vi "Execute.vi"(8 "error in (no error)":errorcluster, 10 "Abstract Consumer in":refnum<class "Abstract Consumer.lvclass">, 11 "Log Close Message in":refnum<class "Log Close Message.lvclass">) -> (0 "error out":errorcluster, 1 "Abstract Response out":refnum<class "Abstract Response Message.lvclass">, 2 "Abstract Consumer out":refnum<class "Abstract Consumer.lvclass">, 3 "Log Close Message out":refnum<class "Log Close Message.lvclass">, 4 "Stop?":bool)   [LabVIEW 2020, in "Log Close Message.lvclass"]
uses:
  Log Close Message.lvclass
  Abstract Log Consumer/Abstract Log Consumer.lvclass
  Consumer/Abstract Consumer/Abstract Consumer.lvclass
  Message/Abstract Response Message/Abstract Response Message.lvclass
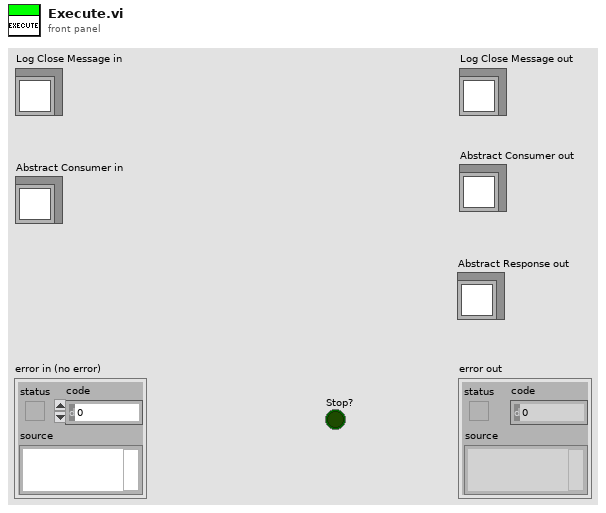
[diagram p1: front panel]
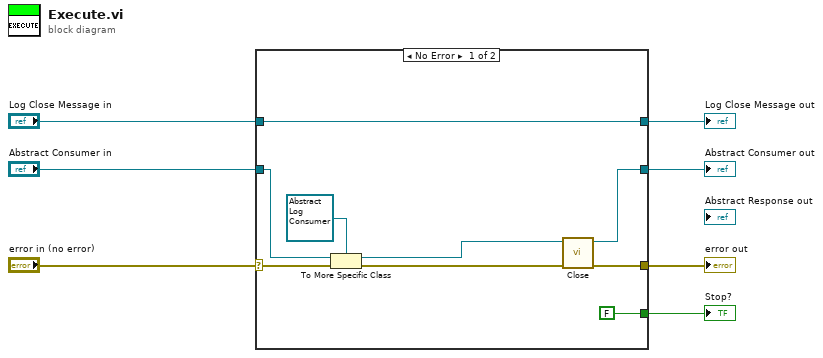
[diagram p0: block diagram]
diagram:
  n1 = case shown="No Error" "error in (no error)" {
    selector: "error in (no error)" -> [w15 w17]
    tunnel: "Abstract Consumer in" -> [w16 w18]
    tunnel: "Log Close Message in" -> [w9 w19]
    tunnel: [w11 w17] -> w4
    tunnel: [w9 w19] -> w2
    tunnel: [w10 w18] -> w1
    tunnel: [FALSE _] -> w3
    frame No Error {
      n2 = To More Specific Class(target class=refnum<class "Abstract Log Consumer.lvclass"> refnum ("Messaging.lvlib:Abstract Log Consumer.lvclass"), reference=w16, error in=w15) -> (specific class reference=w12:refnum<class "Abstract Log Consumer.lvclass">, error out=w13:errorcluster)
      n3 = call-dynamic "Close.vi"("error in (no error)"=w13, "Abstract Log Consumer in"=w12) -> ("error out"=w11:errorcluster, "Abstract Log Consumer out"=w10:refnum<class "Abstract Log Consumer.lvclass">)  [unwired: 8 in]
    }
    frame Error {
    }
  }
  "error out" <- w4
  "Log Close Message out" <- w2
  "Abstract Consumer out" <- w1
  "Stop?" <- w3
